vi "MOKO ExPlugin.vi"() -> ()   [LabVIEW 2018]
uses:
  Lib/STM/Loop/MOKO_ExPlugin_Loop_STM.ctl
  Lib/STM/Loop/MOKO_ExPlugin_Loop_ITEM.ctl
  Lib/STM/Grafic/MOKO_ExPlugin_Grafic_STM.ctl
  Lib/STM/Grafic/MOKO_ExPlugin_Grafic_ITEM.ctl
panel:
  in  "STOP":bool
  out "Waveform Graph":dbl[](graph)
  in  "Reset":bool
  in  "Start":bool
  in  "Stop Graph":bool
  in  "Open SubVi":bool
  in  "Change Led loop":bool
  out "Led loop":bool
  out "Led event":bool
  out "Result":dbl
  in  "Param 2":dbl
  in  "Param 1":dbl
  in  "Sum":bool
  in  "Stop Led":bool
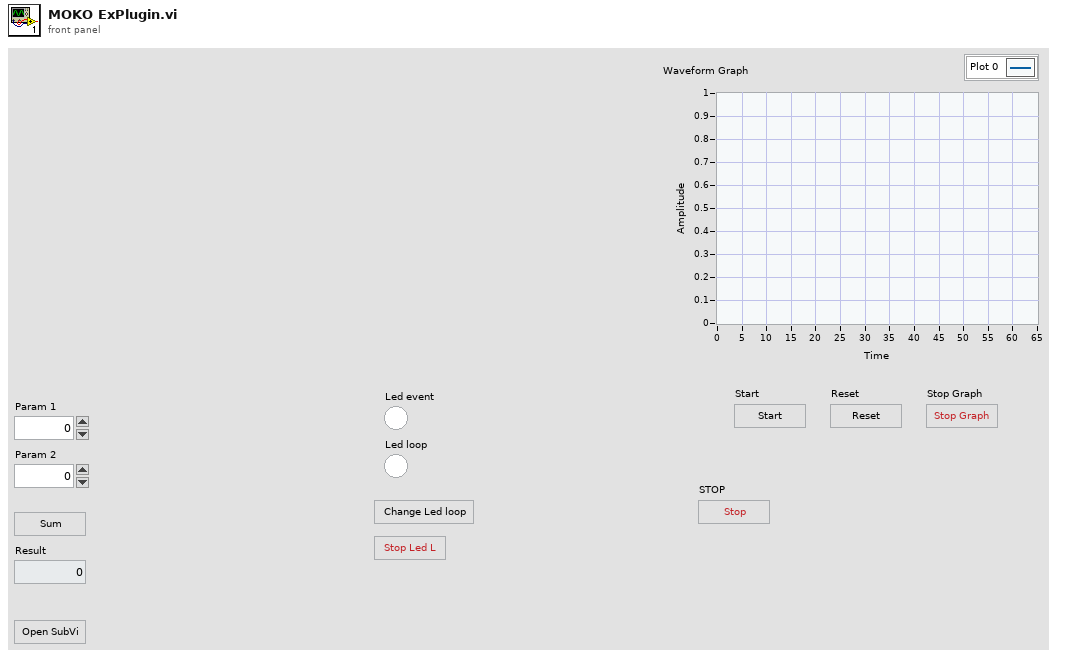
[diagram p1: front panel]
types:
  T1 = typedef "MOKO_ExPlugin_Grafic_STM.ctl" = cluster{"main stm":T2, "data":string}
  T2 = typedef "MOKO_ExPlugin_Grafic_ITEM.ctl" = enum16{"idle", "Write Graph", "Reset", "Start", "Stop", "Stop Graph"}
  T3 = typedef "MOKO_ExPlugin_Loop_STM.ctl" = cluster{"main stm":T4, "data":string}
  T4 = typedef "MOKO_ExPlugin_Loop_ITEM.ctl" = enum16{"idle", "Reset", "Stop", "Sum", "Change LED", "Sync", "Inc", "Led", "OpenSubVi", "Graph"}
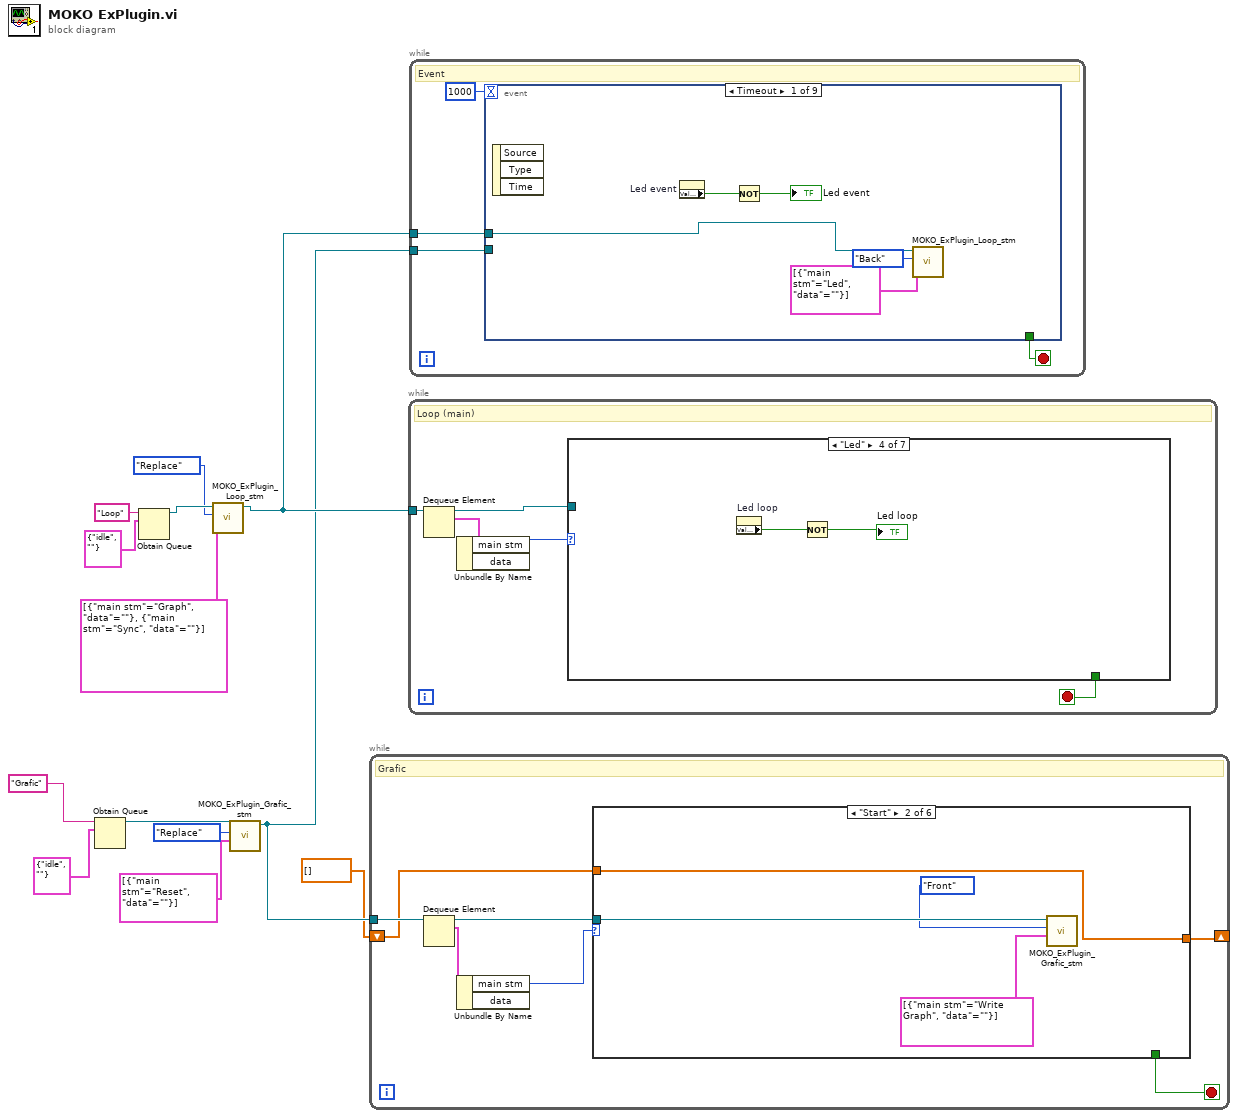
[diagram p0: block diagram]
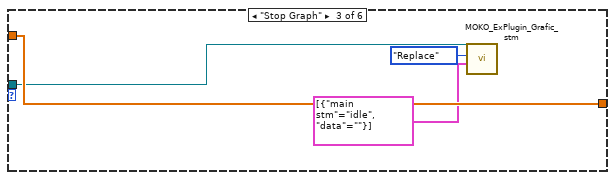
[diagram p3: hidden frame]
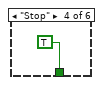
[diagram p4: hidden frame]
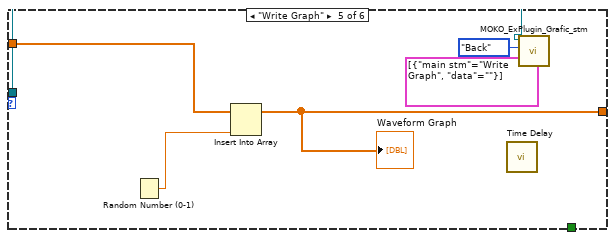
[diagram p5: hidden frame]
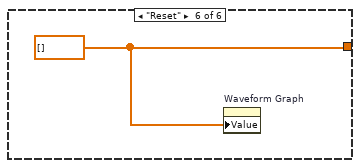
[diagram p6: hidden frame]
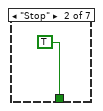
[diagram p8: hidden frame]
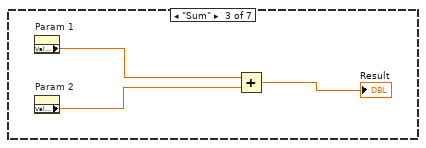
[diagram p9: hidden frame]
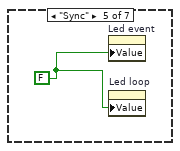
[diagram p10: hidden frame]
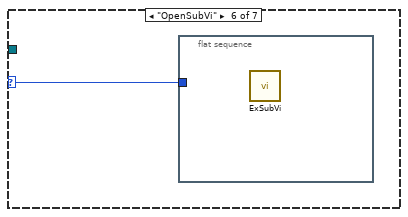
[diagram p11: hidden frame]
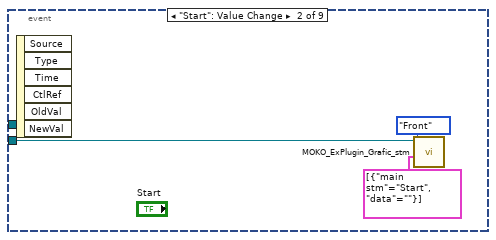
[diagram p13: hidden frame]
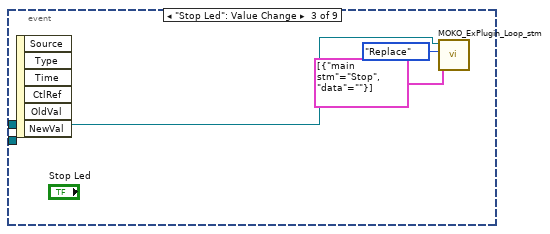
[diagram p14: hidden frame]
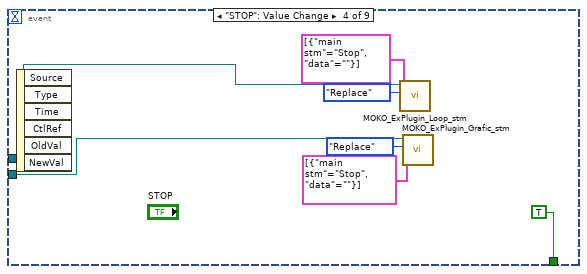
[diagram p15: hidden frame]
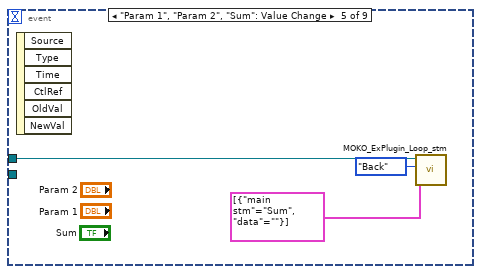
[diagram p16: hidden frame]
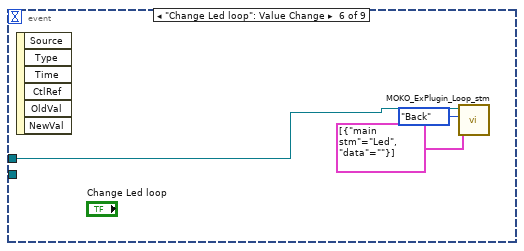
[diagram p17: hidden frame]
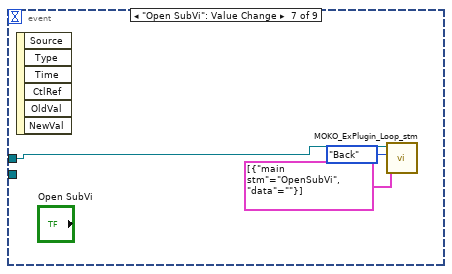
[diagram p18: hidden frame]
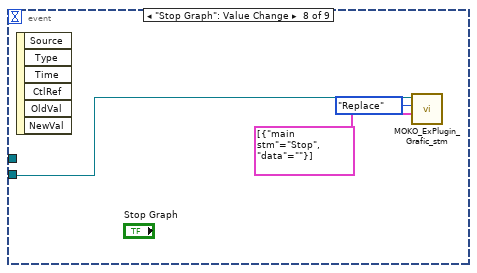
[diagram p19: hidden frame]
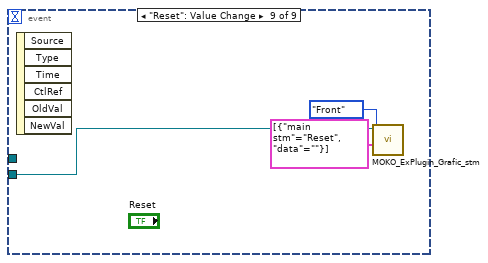
[diagram p20: hidden frame]
diagram:
  n1 = Obtain Queue(name (unnamed)="Grafic", element data type=T1 {"main stm"=enum."idle", "data"=""} ("MOKO_NMEA")) -> (queue out=w4:refnum<queue>)  [unwired: 3 in, 2 out]
  n2 = Obtain Queue(name (unnamed)="Loop", element data type=T3 {"main stm"=enum."idle", "data"=""} ("MOKO_SE_STM")) -> (queue out=w11:refnum<queue>)  [unwired: 3 in, 2 out]
  n3 = call "MOKO_ExPlugin_Loop_stm.vi"("StateMachineSteps"=T3[] [{"main stm"=enum."Graph", "data"=""}, {"main stm"=enum."Sync", "data"=""}], "FNs"=enum16{"Back", "Front", "Replace"}."Replace", "queue in"=w11) -> ("queue out"=w10:refnum<queue>)  [unwired: 7 in, 1 out]
  n4 = call "MOKO_ExPlugin_Grafic_stm.vi"("StateMachineSteps"=T1[] [{"main stm"=enum."Reset", "data"=""}], "FNs"=enum16{"Back", "Front", "Replace"}."Replace", "queue in"=w4) -> ("queue out"=w6:refnum<queue>)  [unwired: 7 in, 1 out]
  n5 = while {
    tunnel: w6 -> [w18]
    shift-right: [w15] -> _
    shift-left: dbl[] [] ("Waveform Graph") -> [w16]
    stop <- w14 stop-if-true
    # "Grafic"
    n6 = Dequeue Element(queue=w18) -> (queue out=w19:refnum<queue>, element=w20:T1)  [unwired: 2 in, 2 out]
    n7 = Unbundle By Name(w20) -> ("main stm"=w17:T2)  [unwired: 1 out]
    n8 = case shown="\"Start\"" w17 {
      tunnel: w19 -> [_ w25 w26 _ w35 _]
      tunnel: w16 -> [w21 w22 w29 _ w33 _]
      tunnel: [w21 w22 w29 _ w31 w37] -> w15
      tunnel: [_ _ _ TRUE _ _] -> w14
      frame "idle", Default {
      }
      frame "Start" {
        n9 = call "MOKO_ExPlugin_Grafic_stm.vi"("StateMachineSteps"=T1[] [{"main stm"=enum."Write Graph", "data"=""}], "FNs"=enum16{"Back", "Front", "Replace"}."Front", "queue in"=w25) -> ()  [unwired: 7 in, 2 out]
      }
      frame "Stop Graph" {
        n10 = call "MOKO_ExPlugin_Grafic_stm.vi"("StateMachineSteps"=T1[] [{"main stm"=enum."idle", "data"=""}], "FNs"=enum16{"Back", "Front", "Replace"}."Replace", "queue in"=w26) -> ()  [unwired: 7 in, 2 out]
      }
      frame "Stop" {
      }
      frame "Write Graph" {
        n11 = Random Number (0-1)() -> (number: 0 to 1=w32:dbl)
        n12 = Insert Into Array(array=w33, new element=w32) -> (w31:dbl[])  [unwired: 1 in]
        "Waveform Graph" <- w31
        n13 = call "Time Delay"() -> ()  [unwired: 11 in, 1 out]
        n14 = call "MOKO_ExPlugin_Grafic_stm.vi"("StateMachineSteps"=T1[] [{"main stm"=enum."Write Graph", "data"=""}], "FNs"=enum16{"Back", "Front", "Replace"}."Back", "queue in"=w35) -> ()  [unwired: 7 in, 2 out]
      }
      frame "Reset" {
        w37 = dbl[] [] ("Waveform Graph")
        n15 = property on="Waveform Graph" class="WFGraph (strict)"("Value"=w37) -> ()  [unwired: 2 in, 2 out]
      }
    }
  }
  n16 = while {
    tunnel: w10 -> [w42]
    stop <- w41 stop-if-true
    # "Loop (main)"
    n17 = Dequeue Element(queue=w42) -> (queue out=w40:refnum<queue>, element=w39:T3)  [unwired: 2 in, 2 out]
    n18 = Unbundle By Name(w39) -> ("main stm"=w38:T4)  [unwired: 1 out]
    n19 = case shown="\"Led\"" w38 {
      selector: w38 -> [_ _ _ _ _ w50 _]
      tunnel: [_ TRUE _ _ _ _ _] -> w41
      tunnel: w40 -> [_ _ _ _ _ _ _]
      frame "idle", Default {
      }
      frame "Stop" {
      }
      frame "Sum" {
        n20 = property on="Param 1" class="DigNum (strict)"() -> ("Value"=w45:dbl)  [unwired: 2 in, 2 out]
        n21 = property on="Param 2" class="DigNum (strict)"() -> ("Value"=w46:dbl)  [unwired: 2 in, 2 out]
        n22 = Add(x=w45, y=w46) -> (x+y=→"Result":dbl)
      }
      frame "Led" {
        n23 = property on="Led loop" class="Bool (strict)"() -> ("Value"=w48:bool)  [unwired: 2 in, 2 out]
        n24 = Not(x=w48) -> (.not. x?=→"Led loop":bool)
      }
      frame "Sync" {
        w49 = FALSE
        n25 = property on="Led event" class="Bool (strict)"("Value"=w49) -> ()  [unwired: 2 in, 2 out]
        n26 = property on="Led loop" class="Bool (strict)"("Value"=w49) -> ()  [unwired: 2 in, 2 out]
      }
      frame "OpenSubVi" {
        n27 = flat-sequence {
          tunnel: w50 -> [_]
          frame #0 {
            n28 = call "ExSubVi.vi"() -> ()  [unwired: 12 in]
          }
        }
      }
      frame "Reset" {
      }
    }
  }
  n29 = while {
    tunnel: w10 -> [w53]
    tunnel: w6 -> [w52]
    stop <- w51 stop-if-true
    # "Event"
    n30 = event shown="[0] Timeout" {
      selector: _ -> [_ _ _ _ _ _ _ _ _]
      dyn-events: _ -> [_ _ _ _ _ _ _ _ _]
      timeout: 1000 -> [_ _ _ _ _ _ _ _ _]
      tunnel: w53 -> [w55 _ w63 w68 w73 w76 w81 _ _]
      tunnel: w52 -> [_ w62 _ w71 _ _ _ w84 w87]
      tunnel: [_ _ _ TRUE _ _ _ _ _] -> w51
      event Timeout {
        n31 = event-data() -> ()  [unwired: 1 in, 3 out]
        n32 = property on="Led event" class="Bool (strict)"() -> ("Value"=w59:bool)  [unwired: 2 in, 2 out]
        n33 = Not(x=w59) -> (.not. x?=→"Led event":bool)
        n34 = call "MOKO_ExPlugin_Loop_stm.vi"("StateMachineSteps"=T3[] [{"main stm"=enum."Led", "data"=""}], "FNs"=enum16{"Back", "Front", "Replace"}."Back", "queue in"=w55) -> ()  [unwired: 7 in, 2 out]
      }
      event "Start": Value Change {
        n35 = event-data() -> ()  [unwired: 1 in, 6 out]
        n36 = call "MOKO_ExPlugin_Grafic_stm.vi"("StateMachineSteps"=T1[] [{"main stm"=enum."Start", "data"=""}], "FNs"=enum16{"Back", "Front", "Replace"}."Front", "queue in"=w62) -> ()  [unwired: 7 in, 2 out]
      }
      event "Stop Led": Value Change {
        n37 = event-data() -> ()  [unwired: 1 in, 6 out]
        n38 = call "MOKO_ExPlugin_Loop_stm.vi"("StateMachineSteps"=T3[] [{"main stm"=enum."Stop", "data"=""}], "FNs"=enum16{"Back", "Front", "Replace"}."Replace", "queue in"=w63) -> ()  [unwired: 7 in, 2 out]
      }
      event "STOP": Value Change {
        n39 = event-data() -> ()  [unwired: 1 in, 6 out]
        n40 = call "MOKO_ExPlugin_Loop_stm.vi"("StateMachineSteps"=T3[] [{"main stm"=enum."Stop", "data"=""}], "FNs"=enum16{"Back", "Front", "Replace"}."Replace", "queue in"=w68) -> ()  [unwired: 7 in, 2 out]
        n41 = call "MOKO_ExPlugin_Grafic_stm.vi"("StateMachineSteps"=T1[] [{"main stm"=enum."Stop", "data"=""}], "FNs"=enum16{"Back", "Front", "Replace"}."Replace", "queue in"=w71) -> ()  [unwired: 7 in, 2 out]
      }
      event "Param 1", "Param 2", "Sum": Value Change {
        n42 = event-data() -> ()  [unwired: 1 in, 6 out]
        n43 = call "MOKO_ExPlugin_Loop_stm.vi"("StateMachineSteps"=T3[] [{"main stm"=enum."Sum", "data"=""}], "FNs"=enum16{"Back", "Front", "Replace"}."Back", "queue in"=w73) -> ()  [unwired: 7 in, 2 out]
      }
      event "Change Led loop": Value Change {
        n44 = event-data() -> ()  [unwired: 1 in, 6 out]
        n45 = call "MOKO_ExPlugin_Loop_stm.vi"("StateMachineSteps"=T3[] [{"main stm"=enum."Led", "data"=""}], "FNs"=enum16{"Back", "Front", "Replace"}."Back", "queue in"=w76) -> ()  [unwired: 7 in, 2 out]
      }
      event "Open SubVi": Value Change {
        n46 = event-data() -> ()  [unwired: 1 in, 6 out]
        n47 = call "MOKO_ExPlugin_Loop_stm.vi"("StateMachineSteps"=T3[] [{"main stm"=enum."OpenSubVi", "data"=""}], "FNs"=enum16{"Back", "Front", "Replace"}."Back", "queue in"=w81) -> ()  [unwired: 7 in, 2 out]
      }
      event "Stop Graph": Value Change {
        n48 = event-data() -> ()  [unwired: 1 in, 6 out]
        n49 = call "MOKO_ExPlugin_Grafic_stm.vi"("StateMachineSteps"=T1[] [{"main stm"=enum."Stop", "data"=""}], "FNs"=enum16{"Back", "Front", "Replace"}."Replace", "queue in"=w84) -> ()  [unwired: 7 in, 2 out]
      }
      event "Reset": Value Change {
        n50 = event-data() -> ()  [unwired: 1 in, 6 out]
        n51 = call "MOKO_ExPlugin_Grafic_stm.vi"("StateMachineSteps"=T1[] [{"main stm"=enum."Reset", "data"=""}], "FNs"=enum16{"Back", "Front", "Replace"}."Front", "queue in"=w87) -> ()  [unwired: 7 in, 2 out]
      }
    }
  }
